vi "Interface.vi"() -> ()   [LabVIEW 2023]
panel:
  out "read buffer":string
  in  "Arduino Load Cell Readings?":refnum<visa-resource-name>
  in  "Frequency":dbl
  in  "VISA resource name":refnum<visa-resource-name>
  in  "number of times to repeat":string caption="n"
  in  "desired strain %":dbl
  in  "sample length (mm)":dbl
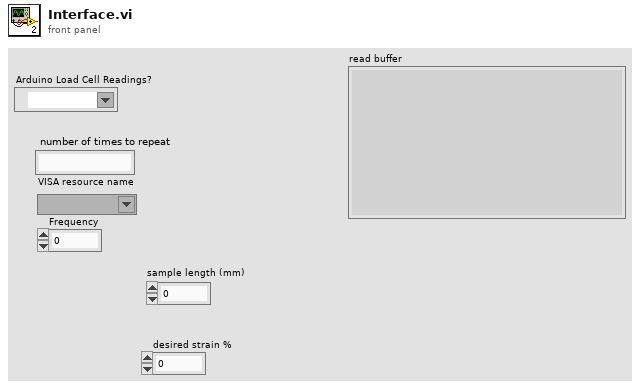
[diagram p1: front panel]
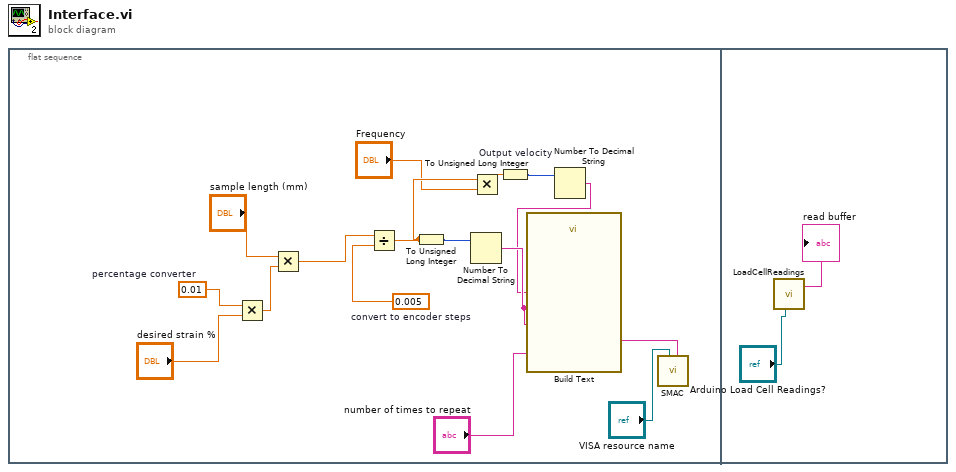
[diagram p0: block diagram]
diagram:
  n1 = flat-sequence {
    frame #0 {
      w11 = 0.005  # convert to encoder steps
      w14 = 0.01  # percentage converter
      n2 = Multiply(x=w14, y="desired strain %") -> (x*y=w13:dbl)
      n3 = Multiply(x="sample length (mm)", y=w13) -> (x*y=w12:dbl)
      n4 = Divide(x=w12, y=w11) -> (x/y=w5:dbl)
      n5 = To Unsigned Long Integer(number=w5) -> (unsigned 32bit integer=w10:u32)
      n6 = Number To Decimal String(number=w10) -> (decimal integer string=w7:string)  [unwired: 1 in]
      n7 = Multiply(x=w5, y="Frequency") -> (x*y=w3:dbl)
      n8 = To Unsigned Long Integer "Output velocity"(number=w3) -> (unsigned 32bit integer=w9:u32)
      n9 = Number To Decimal String(number=w9) -> (decimal integer string=w6:string)  [unwired: 1 in]
      n10 = call "Build Text"("n"="number of times to repeat", "vel"=w6, "counts"=w7, "counts2"=w7) -> ("Result"=w2:string)  [unwired: 10 in, 1 out]
      n11 = call "SMAC.vi"("write buffer"=w2, "VISA resource name"="VISA resource name") -> ()  [unwired: 10 in]
    }
    frame #1 {
      n12 = call "LoadCellReadings.vi"("Arduino Load Cell Readings?"="Arduino Load Cell Readings?") -> ("read buffer"=→"read buffer":string)  [unwired: 10 in]
    }
  }
